vi "Elapse or Normal Time and Format.vi"(10 "Elapsed?":bool, 11 "Time Array":timestamp[](array[timestamp])) -> (2 "Time Array":dbl[](array[numeric]), 3 "X Scale.Display Format:Format":u8)   [LabVIEW 2023]
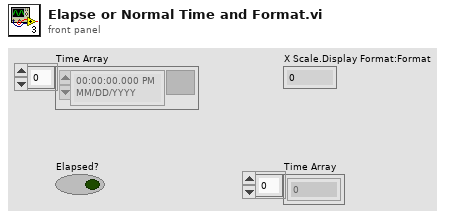
[diagram p1: front panel]
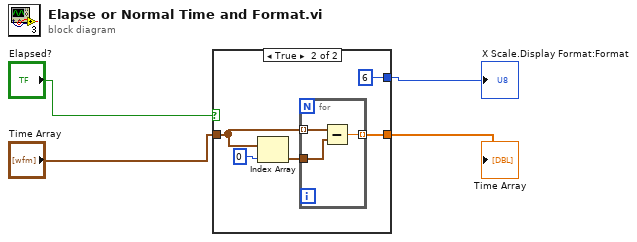
[diagram p0: block diagram]
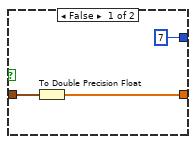
[diagram p2: hidden frame]
diagram:
  n1 = case shown="True" "Elapsed?" {
    tunnel: "Time Array" -> [w7 w11]
    tunnel: [w6 w9] -> w3
    tunnel: [u8 7 ("X Scale.Display Format:Format") u8 6 ("X Scale.Display Format:Format")] -> w2
    frame False {
      n2 = To Double Precision Float(number=w7) -> (double precision float=w6:dbl[])
    }
    frame True {
      n3 = Index Array(array=w11, index=0) -> (element=w10:timestamp)
      n4 = for {
        tunnel: w11 -> [w15] mode=indexing
        tunnel: w10 -> [w14]
        tunnel: [w13] -> w9 mode=indexing
        n5 = Subtract(x=w15, y=w14) -> (x-y=w13:dbl)
      }
    }
  }
  "Time Array" <- w3
  "X Scale.Display Format:Format" <- w2
